vi "REV Rotations to Degrees.vi"(11 "Steer Angles (rotations)":T1) -> (3 "Steer Angles (degrees)":T1)   [LabVIEW 2020]
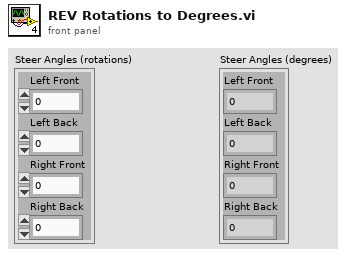
[diagram p1: front panel]
types:
  T1 = cluster{"Left Front":dbl, "Left Back":dbl, "Right Front":dbl, "Right Back":dbl}
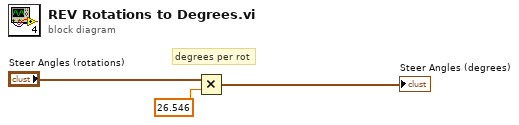
[diagram p0: block diagram]
diagram:
  # "degrees per rot"
  n1 = Multiply(x="Steer Angles (rotations)", y=26.546) -> (x*y=→"Steer Angles (degrees)":T1)
